vi "set_ai_noise_filter.vi"(8 "error in (no error)":errorcluster, 10 "Line frequency":enum16{"60 Hz", "50 Hz"}(ring), 11 "Modbus Master in":refnum<class "Modbus Master.lvclass">) -> (0 "error out":errorcluster, 3 "Modbus Master out":refnum<class "Modbus Master.lvclass">)   [LabVIEW 2018, in "ICP xET-7017.lvlib"]
uses:
  <vilib>/NI/Modbus Library/API/Master/Modbus Master.lvclass
  ICP xET-7017.lvlib
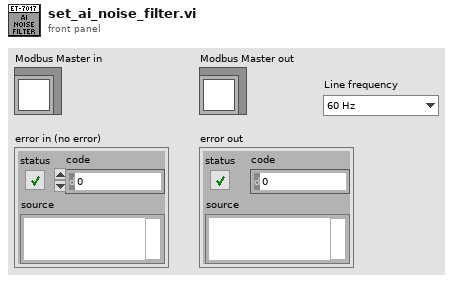
[diagram p1: front panel]
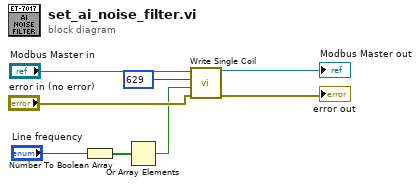
[diagram p0: block diagram]
diagram:
  n1 = Number To Boolean Array(number="Line frequency") -> (Boolean array=w3:bool[])
  n2 = Or Array Elements(Boolean array=w3) -> (logical OR=w1:bool)
  n3 = call-dynamic "Write Single Coil.vi"("error in"="error in (no error)", "coil to write"=w1, "address"=u16 629 ("starting address"), "Modbus master in"="Modbus Master in") -> ("error out"=→"error out":errorcluster, "Modbus master out"=→"Modbus Master out":refnum<class "Modbus Master.lvclass">)  [unwired: 6 in]
